vi "Parse Heartbeat.vi"(8 "error in":errorcluster, 10 "Hearbeat in":u8[](array[numeric]), 11 "Kronos in":refnum<class "Kronos.lvclass">) -> (0 "error out":errorcluster, 3 "Kronos out":refnum<class "Kronos.lvclass">)   [LabVIEW 2018, in "Kronos.lvlib" / "Kronos.lvclass"]
uses:
  Kronos.lvclass
  Custom Controls/Heartbeat Status.ctl
  Kronos.lvclass/Kronos.ctl
  Kronos.lvlib
  builds/Laser.lvlibp/Laser.lvclass
  C:/Users/Ron.Dexter.LUMINARTECH/Desktop/builds/Laser.lvlibp/Laser.lvclass
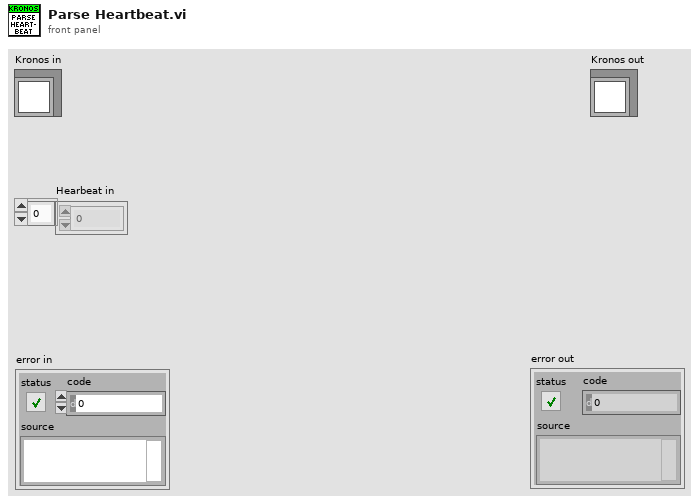
[diagram p1: front panel]
types:
  T1 = typedef "Kronos.lvlib/Heartbeat Status.ctl" = cluster{"Laser Status":bool, "On Time":dbl, "State":string, "Input Voltage":dbl, "Case Temp °C":dbl, "Board Temp °C":dbl, "Seed Temp °C":dbl, "PumpTemp °C":dbl, "Pulse Frequency (Hz)":u32, "Output Power (mW)":dbl}
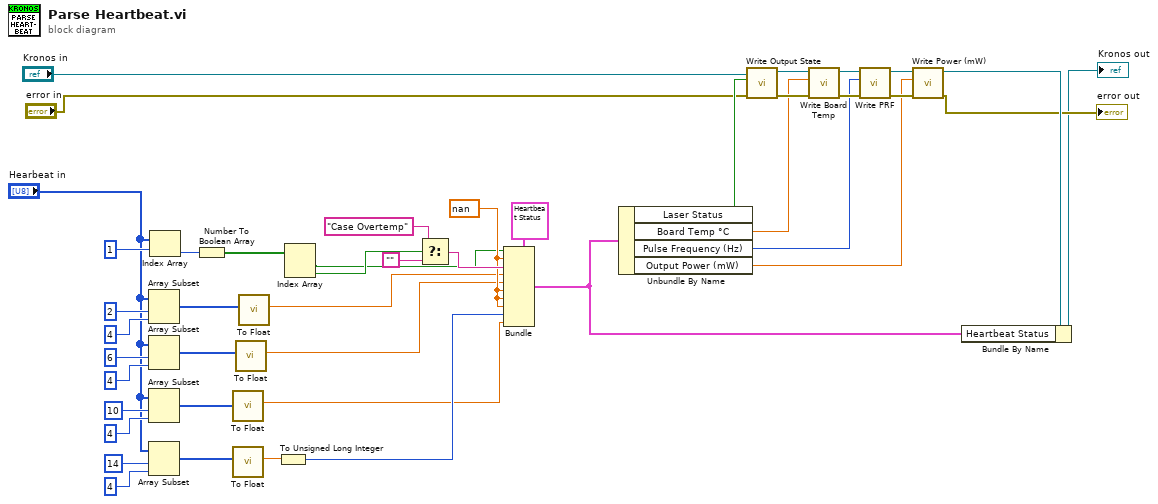
[diagram p0: block diagram]
diagram:
  w21 = nan ("On Time:")
  n1 = Array Subset(array="Hearbeat in", index=2, length=4) -> (w22:u8[])
  n2 = Array Subset(array="Hearbeat in", index=6, length=4) -> (w23:u8[])
  n3 = Array Subset(array="Hearbeat in", index=10, length=4) -> (w24:u8[])
  n4 = Array Subset(array="Hearbeat in", index=14, length=4) -> (w27:u8[])
  n5 = Index Array(array="Hearbeat in", index=1) -> (element=w31:u8)
  n6 = Number To Boolean Array(number=w31) -> (Boolean array=w30:bool[])
  n7 = call "To Float.vi"("Status Message"=w24) -> ("Float"=w20:dbl)  [unwired: 10 in]
  n8 = call "To Float.vi"("Status Message"=w27) -> ("Float"=w26:dbl)  [unwired: 10 in]
  n9 = call "To Float.vi"("Status Message"=w23) -> ("Float"=w18:dbl)  [unwired: 10 in]
  n10 = call "To Float.vi"("Status Message"=w22) -> ("Float"=w19:dbl)  [unwired: 10 in]
  n11 = To Unsigned Long Integer(number=w26) -> (unsigned 32bit integer=w25:u32)
  n12 = Index Array(array=w30) -> (element #1=w17:bool, element #2=w29:bool)  [unwired: 2 in]
  n13 = Select(t="Case Overtemp", s=w29, f="") -> (s? t:f=w28:string)
  n14 = Bundle(cluster=T1 {"Laser Status"=FALSE, "On Time"=0.0, "State"="", "Input Voltage"=0.0, "Case Temp °C"=0.0, "Board Temp °C"=0.0, "Seed Temp °C"=0.0, "PumpTemp °C"=0.0, "Pulse Frequency (Hz)"=0, "Output Power (mW)"=0.0} ("Heartbeat Status"), "Laser Status"=w17, "On Time"=w21, "State"=w28, "Input Voltage"=w19, "Case Temp °C"=w18, "Board Temp °C"=w21, "Seed Temp °C"=w21, "PumpTemp °C"=w21, "Pulse Frequency (Hz)"=w25, "Output Power (mW)"=w20) -> (w1:T1)
  n15 = Unbundle By Name(w1) -> ("Laser Status"=w15:bool, "Board Temp °C"=w5:dbl, "Pulse Frequency (Hz)"=w4:u32, "Output Power (mW)"=w3:dbl)
  n16 = call "Write Output State.vi"("error in (no error)"="error in", "Output State"=w15, "Laser in"="Kronos in") -> ("error out"=w10:errorcluster, "Laser out"=w14:refnum<class "Kronos.lvclass">)  [unwired: 7 in]
  n17 = call "Write Board Temp.vi"("error in (no error)"=w10, "Board Temp"=w5, "Laser in"=w14) -> ("error out"=w9:errorcluster, "Laser out"=w13:refnum<class "Kronos.lvclass">)  [unwired: 7 in]
  n18 = call "Write PRF.vi"("error in (no error)"=w9, "PRF"=w4, "Laser in"=w13) -> ("error out"=w8:errorcluster, "Laser out"=w12:refnum<class "Kronos.lvclass">)  [unwired: 7 in]
  n19 = call "Write Power (mW).vi"("error in (no error)"=w8, "Power (mW)"=w3, "Laser in"=w12) -> ("error out"=→"error out":errorcluster, "Laser out"=w11:refnum<class "Kronos.lvclass">)  [unwired: 7 in]
  n20 = Bundle By Name(cluster=w11, "Heartbeat Status"=w1) -> (→"Kronos out":refnum<class "Kronos.lvclass">)
